vi "SVT Sound Level.vi"   [LabVIEW 2017, in "SoundVib_SoundLevel.lvlib"]
doc: "Computes several sound level measurements including equivalent continuous level (Leq), running Leq sound levels, exponential averaged sound level, and the peak sound level. Wire data to the <B>scaled signal [EU]</B> input to determine the polymorphic instance to use or manually select the instance."
uses:
  <vilib>/addons/Sound and Vibration/svt_Level/SoundVib_SoundLevel.lvlib
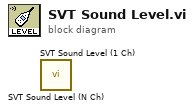
[diagram p0: block diagram]
diagram:
  n1 = call <vilib>:"SVT Sound Level (N Ch).vi"() -> ()  [unwired: 10 in, 6 out]
  n2 = call <vilib>:"SVT Sound Level (1 Ch).vi"() -> ()  [unwired: 10 in, 6 out]
